vi "Parse Input.vi"(11 "Input":string) -> (2 "Boards":i32[][][](array[numeric]), 3 "Draw":i32[](array[numeric]))   [LabVIEW 2021]
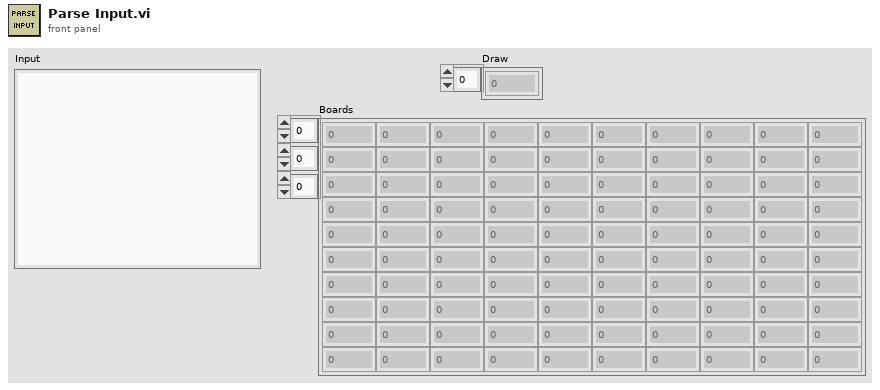
[diagram p1: front panel]
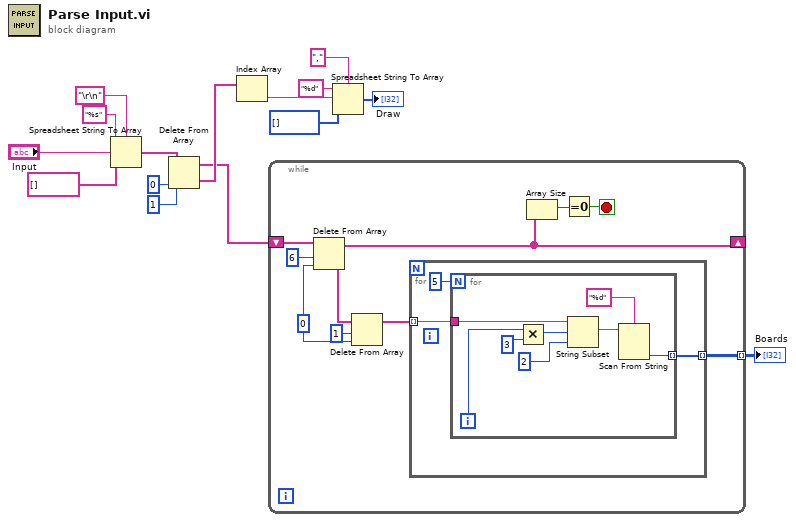
[diagram p0: block diagram]
diagram:
  n1 = Spreadsheet String To Array(delimiter (Tab)="\r\n", format string="%s", spreadsheet string="Input", array type (2D Dbl)=string[] []) -> (array=w12:string[])
  n2 = Delete From Array(array=w12, length=1, index=0) -> (deleted portion=w4:string[], array with subset deleted=w2:string[])
  n3 = Index Array(array=w4) -> (element=w9:string)  [unwired: 1 in]
  n4 = while {
    shift-right: [w20] -> _
    shift-left: w2 -> [w25]
    tunnel: [w17] -> w3 mode=indexing
    stop <- w18 stop-if-true
    w16 = 0 ("index")
    n5 = Delete From Array(array=w25, length=6, index=w16) -> (deleted portion=w23:string[], array with subset deleted=w20:string[])
    n6 = Delete From Array(array=w23, length=1, index=w16) -> (array with subset deleted=w21:string[])  [unwired: 1 out]
    n7 = for {
      tunnel: w21 -> [w28] mode=indexing
      tunnel: [w27] -> w17 mode=indexing
      n8 = for {
        N: 5 -> [_]
        tunnel: w28 -> [w36]
        tunnel: [w29] -> w27 mode=indexing
        i -> [w33]
        n9 = Multiply(x=w33, y=3 ("length (rest)")) -> (x*y=w34:i32)
        n10 = String Subset(string=w36, offset (0)=w34, length (rest)=2 ("length (rest)")) -> (substring=w31:string)
        n11 = Scan From String(format string="%d", input string=w31) -> (output 1=w29:i32)  [unwired: 3 in, 3 out]
      }
    }
    n12 = Array Size(array=w20) -> (size(s)=w19:i32)
    n13 = Equal To 0?(x=w19) -> (x = 0?=w18:bool)
  }
  "Boards" <- w3
  n14 = Spreadsheet String To Array(delimiter (Tab)="," ("format string"), format string="%d", spreadsheet string=w9, array type (2D Dbl)=i32[] []) -> (array=→"Draw":i32[])
